vi "ZCR Find state by thresholds_temp.vi"(10 "Noise amplitude":dbl format="%.2p", 11 "Input Signal":waveform(dbl)[](graph)=[{"t0"=timestamp(3810040522.776 s since 1904-01-01), "dt"=0.0002, "Y"=array[5000 elements]}, {"t0"=timestamp(3810040522.777 s since 1904-01-01), "dt"=0.0002, "Y"=array[5000 elements]}]) -> (2 "SIN OFF Points":i32[](array[numeric]), 3 "SIN ON Points":i32[](array[numeric]))   [LabVIEW 2020, in "Library Commun.lvlib" / "Nodon_ZCR.lvclass"]
uses:
  Nodon_ZCR.lvclass
  <vilib>/Utility/miscctls.llb/LVRangeTypeDef.ctl
  <vilib>/measure/NI_MABase.lvlib
  <vilib>/Analysis/NI_AALPro.lvlib
panel:
  out "Graphe":dbl[](graph)
  in  "Point for zoom":i32
  out "Input Signal":waveform(dbl)[](graph)=[{"t0"=timestamp(3810040522.776 s since 1904-01-01), "dt"=0.0002, "Y"=array[5000 elements]}, {"t0"=timestamp(3810040522.777 s since 1904-01-01), "dt"=0.0002, "Y"=array[5000 elements]}]
  # "This VI Find the ON states and the OFF states based on a fix value\nNot to be used of ZCR control, due to the thresholds noise close to 0"
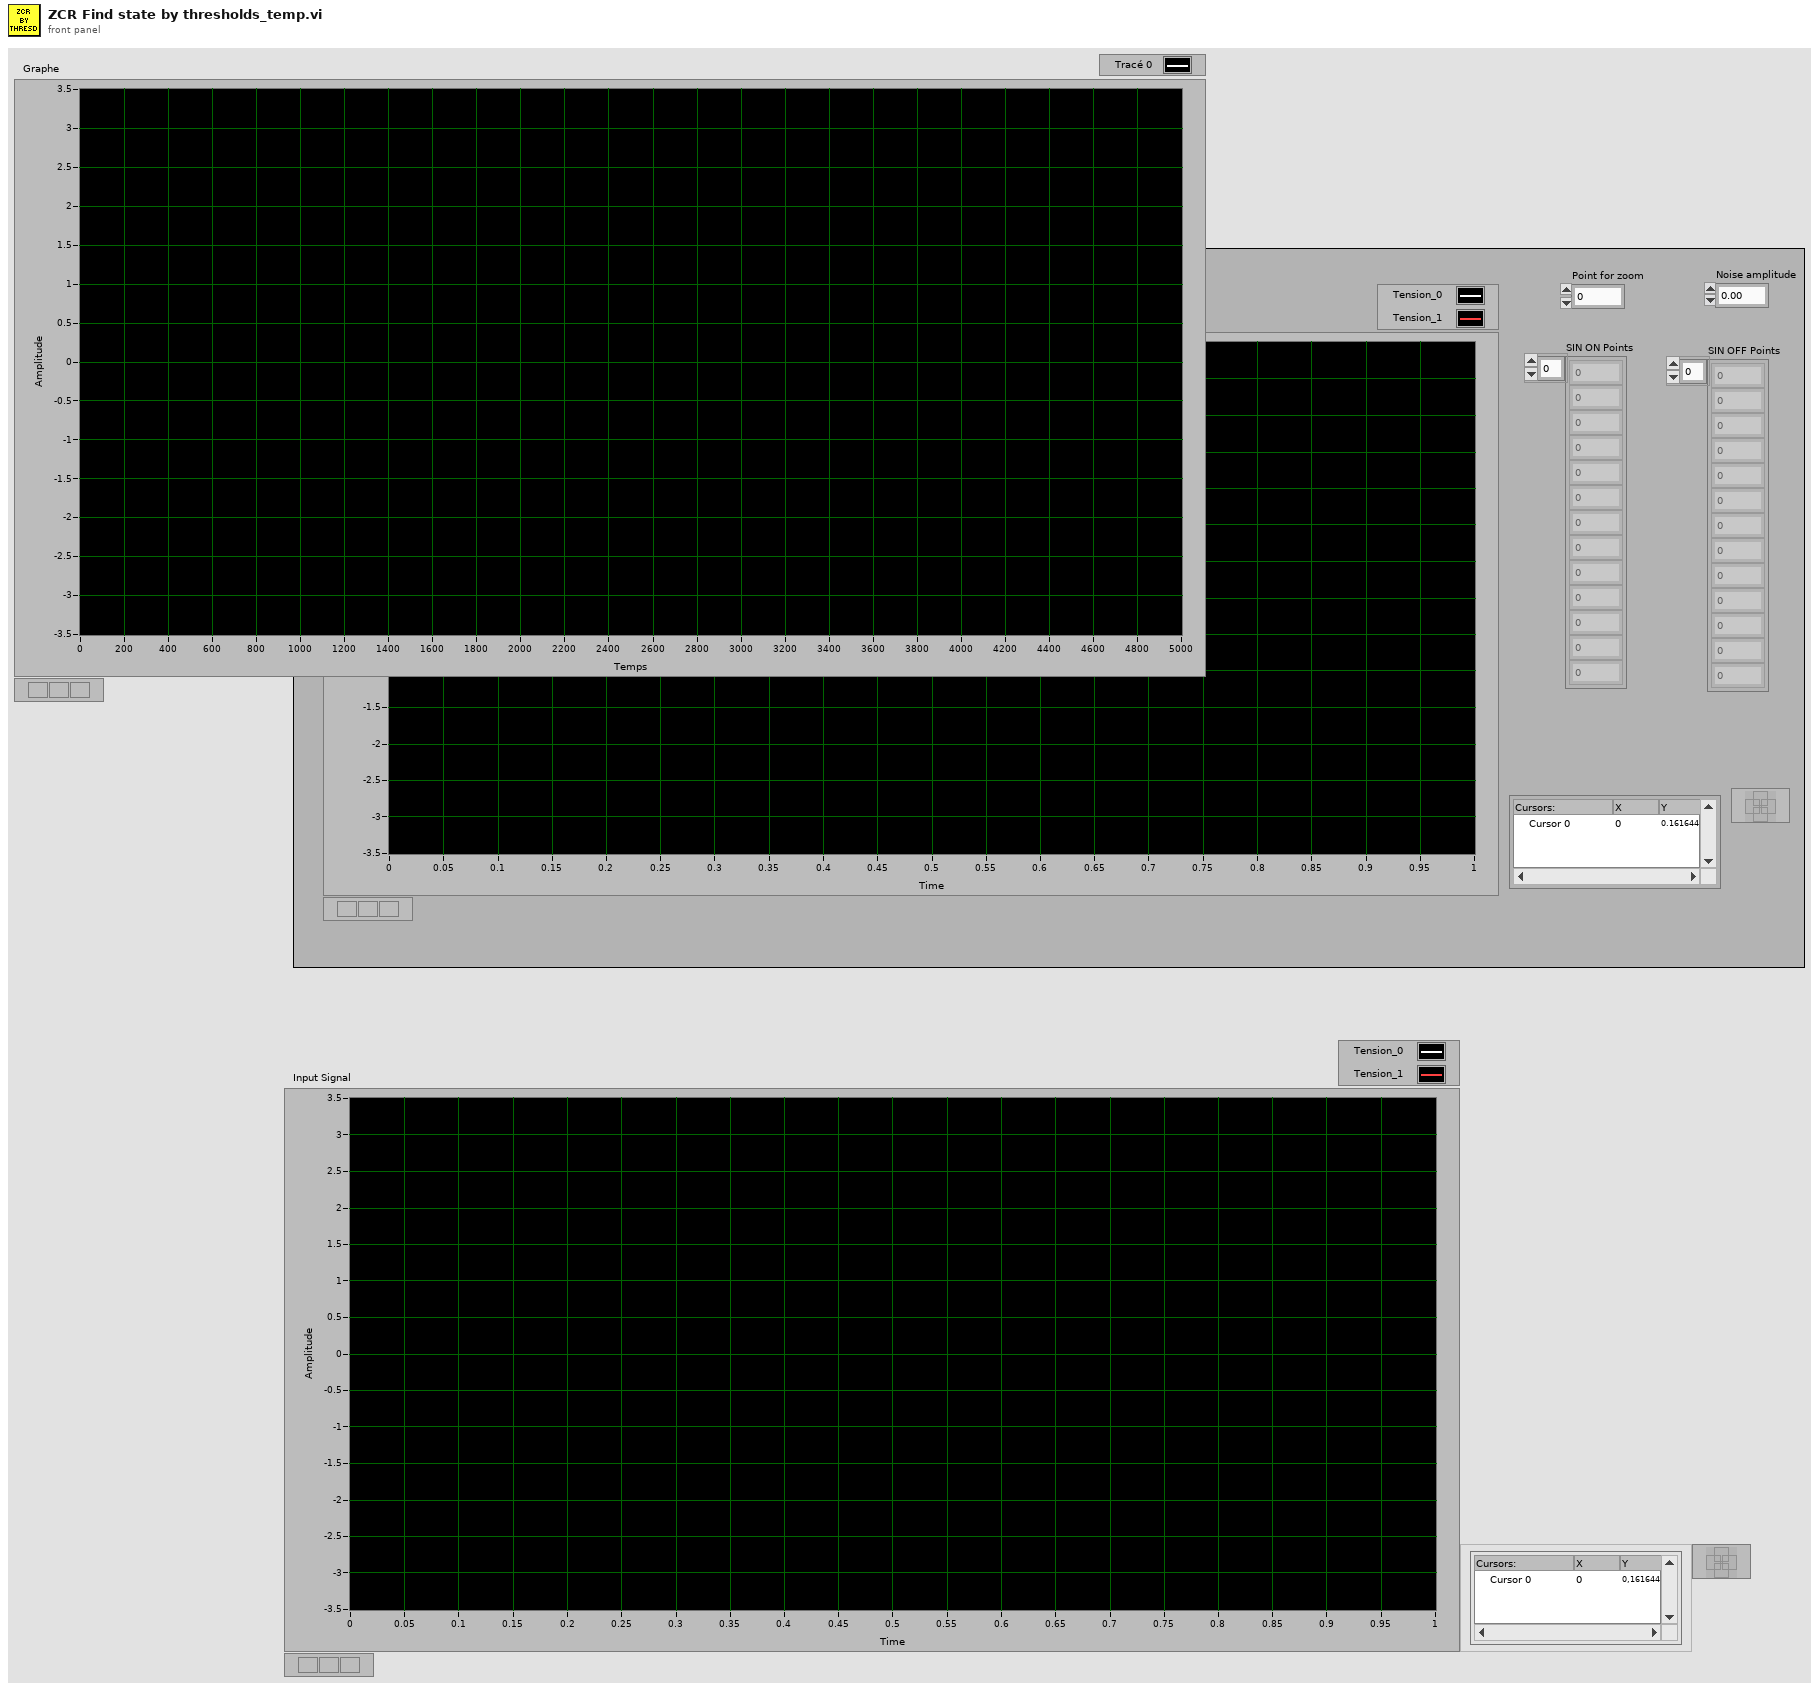
[diagram p1: front panel]
types:
  T1 = typedef "LVRangeTypeDef.ctl" = cluster{"Minimum":dbl, "Maximum":dbl, "Increment":dbl, "Minor Increment":dbl, "Start":dbl}
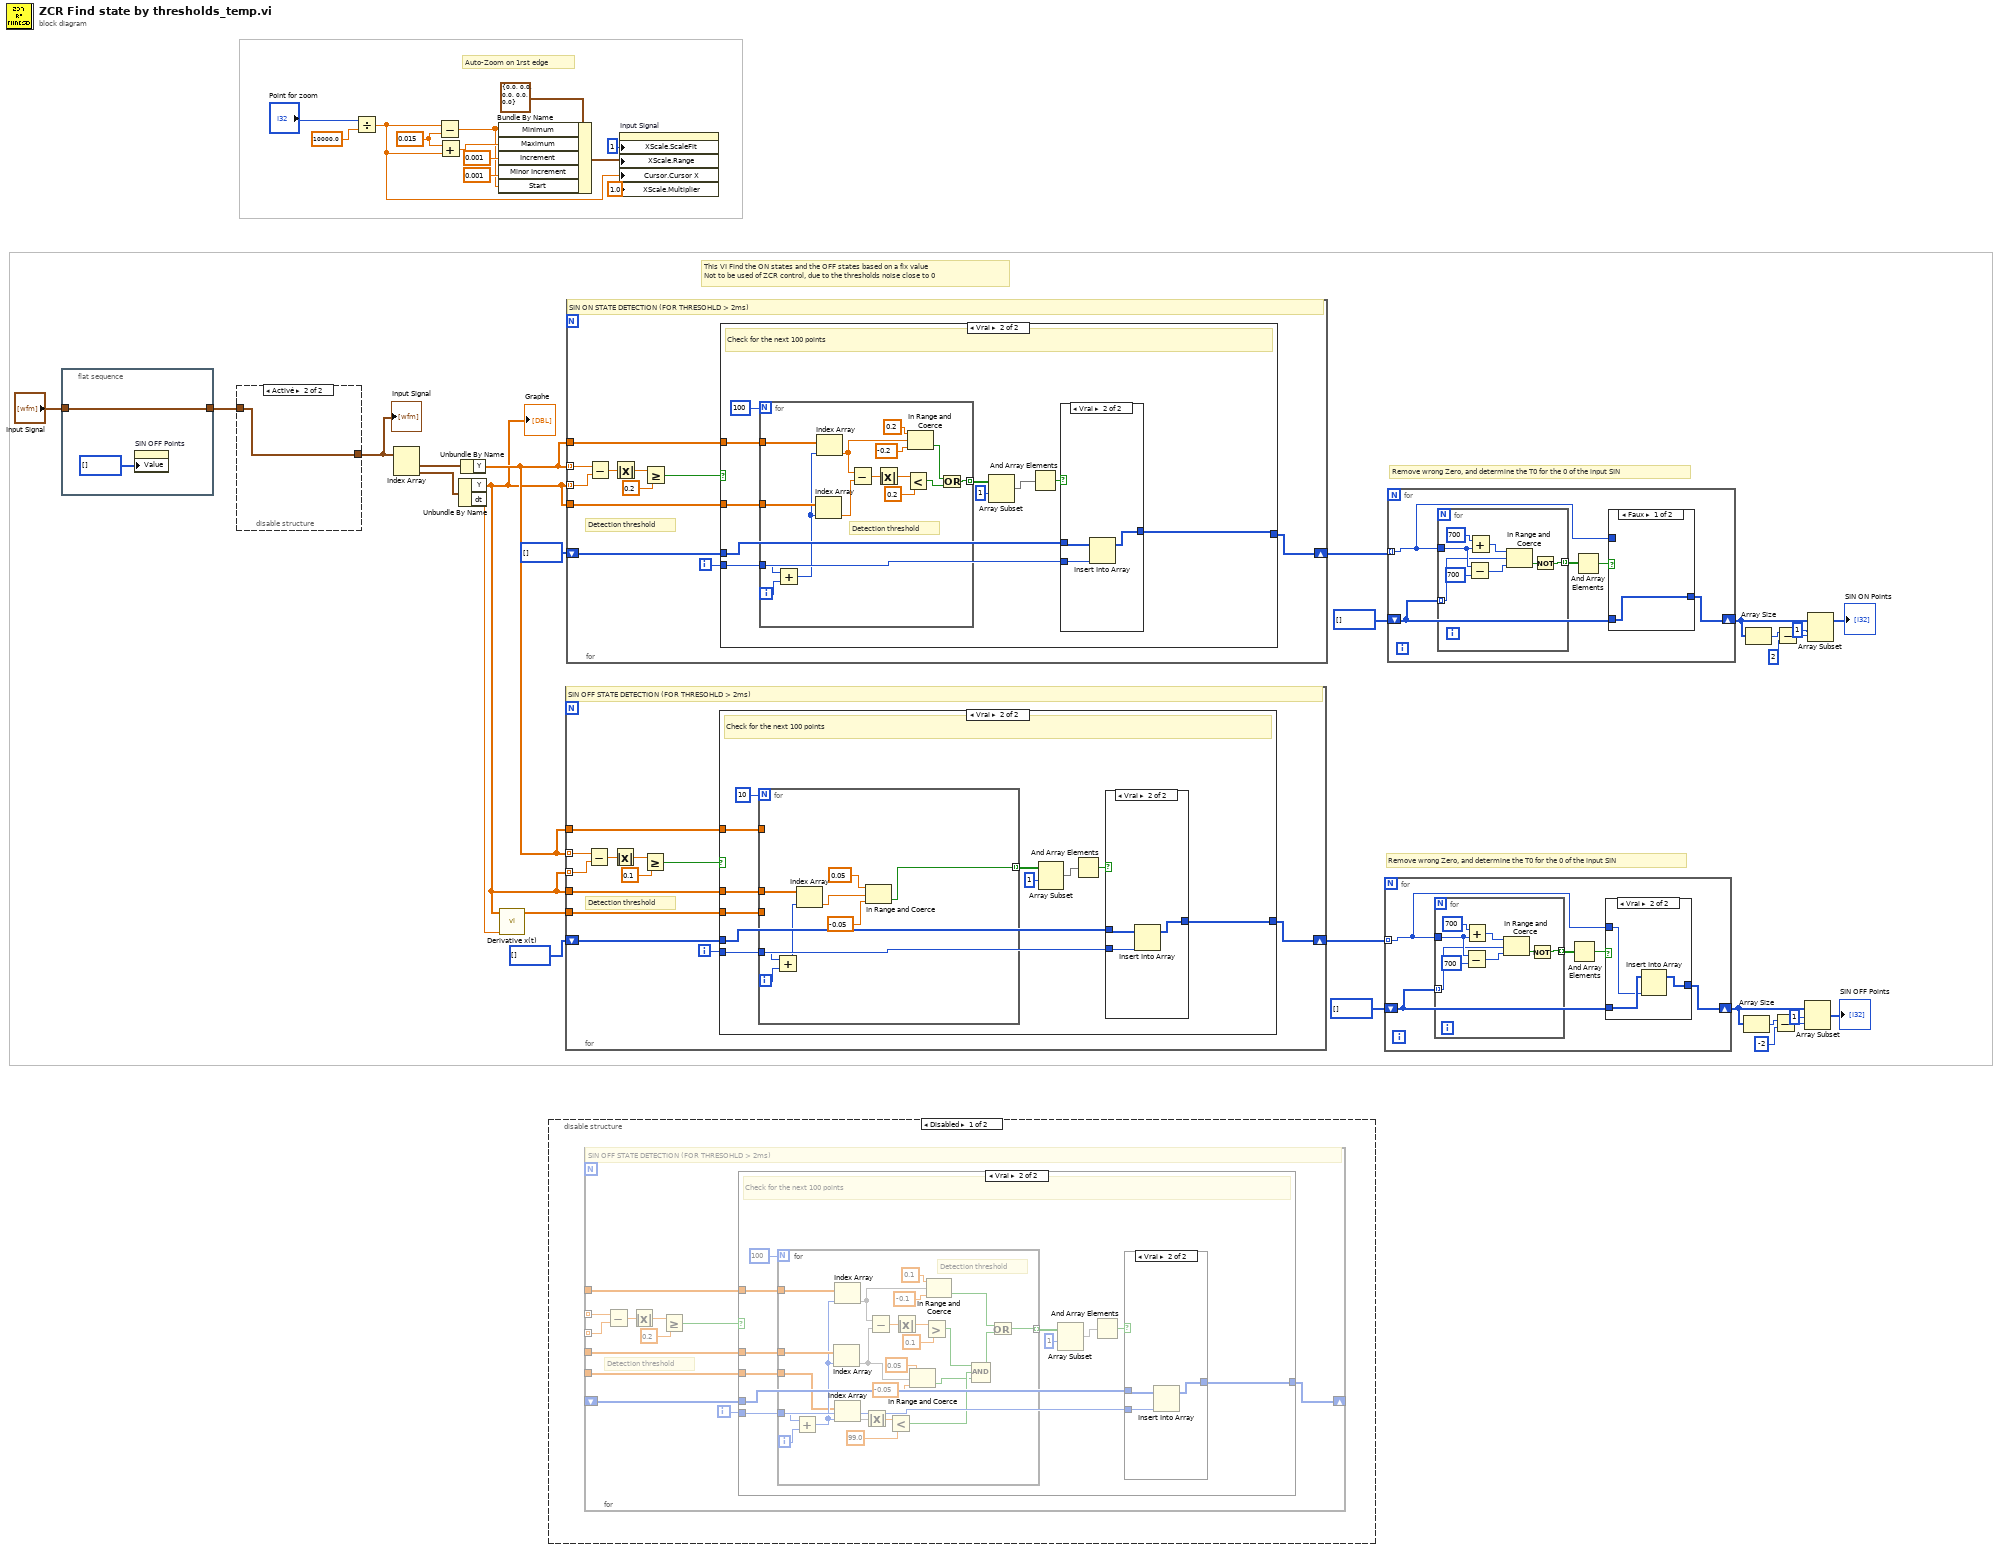
[diagram p0: block diagram]
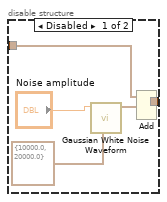
[diagram p2: hidden frame]
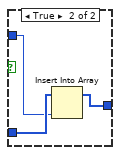
[diagram p6: hidden frame]
diagram:
  w34 = 0.015
  # "Remove wrong Zero, and determine the T0 for the 0 of the input SIN"
  # "Remove wrong Zero, and determine the T0 for the 0 of the input SIN"
  # "This VI Find the ON states and the OFF states based on a fix value\nNot to be used of ZCR control, due to the thresholds noise close to 0"
  # "Auto-Zoom on 1rst edge"
  n1 = flat-sequence {
    tunnel: "Input Signal" -> [w40]
    tunnel: [w40] -> w7
    frame #0 {
      n2 = property on="SIN OFF Points" class="Tabl (strict)"("Value"=i32[] []) -> ()  [unwired: 2 in, 2 out]
    }
  }
  n3 = disable-structure shown="Activé" {
    disable-tunnel: [w44 w47] -> w39
    disable-tunnel: w7 -> [w42 w47]
    frame Disabled {
      n4 = call <vilib>:"Gaussian White Noise Waveform.vi"("sampling info"=cluster{"Fs":dbl, "#s":dbl} {"Fs"=10000.0, "#s"=20000.0}, "standard deviation"="Noise amplitude") -> ("signal out"=w45:waveform(dbl))  [unwired: 8 in, 1 out]
      n5 = Add(1:w45, 2:w42) -> (0:w44:waveform(dbl)[])  [unwired: 1 in, 1 out]
    }
    frame Enabled {
    }
  }
  "Input Signal" <- w39
  n6 = Divide(x="Point for zoom", y=10000.0) -> (x/y=w25:dbl)
  n7 = Index Array(array=w39) -> (element #1=w38:waveform(dbl), element #2=w37:waveform(dbl))  [unwired: 2 in]
  n8 = Subtract(x=w25, y=w34) -> (x-y=w29:dbl)
  n9 = Add(x=w34, y=w25) -> (x+y=w32:dbl)
  n10 = Unbundle By Name(w37) -> ("Y"=w1:dbl[], "dt"=w3:dbl)
  "Graphe" <- w1
  n11 = Unbundle By Name(w38) -> ("Y"=w2:dbl[])
  n12 = Bundle By Name(cluster=T1 {"Minimum"=0.0, "Maximum"=0.0, "Increment"=0.0, "Minor Increment"=0.0, "Start"=0.0} ("X Scale.Range"), "Minimum"=w29, "Maximum"=w32, "Increment"=0.001, "Minor Increment"=0.001, "Start"=w29) -> (w28:T1)
  n13 = call <vilib>:"Derivative x(t).vi"("dt"=w3, "X"=w1) -> ("dX/dt"=w6:dbl[])  [unwired: 8 in, 1 out]
  n14 = disable-structure shown="Disabled" {
    frame Disabled {
      n15 = for {
        tunnel: _ -> [w59] mode=indexing
        tunnel: _ -> [w58] mode=indexing
        shift-right: [w51] -> _
        shift-left: _ -> [w53]
        tunnel: _ -> [w50]
        tunnel: _ -> [w49]
        tunnel: _ -> [w48]
        i -> [w52]
        # "Detection threshold"
        # "SIN OFF STATE DETECTION (FOR THRESOHLD > 2ms)"
        n16 = Subtract(x=w59, y=w58) -> (x-y=w57:dbl)
        n17 = Absolute Value(x=w57) -> (abs(x)=w56:dbl)
        n18 = Greater Or Equal?(x=w56, y=0.2) -> (x >= y?=w54:bool)
        n19 = case shown="Vrai" w54 {
          tunnel: w53 -> [w60 w67]
          tunnel: w52 -> [_ w66]
          tunnel: [w60 w65] -> w51
          tunnel: w50 -> [_ w69]
          tunnel: w49 -> [_ w70]
          tunnel: w48 -> [_ w61]
          frame False {
          }
          frame True {
            # "Check for the next 100 points"
            n20 = for {
              N: 100 -> [_]
              tunnel: w70 -> [w99]
              tunnel: w69 -> [w98]
              tunnel: w66 -> [w94]
              tunnel: [w84] -> w64 mode=indexing
              tunnel: w61 -> [w81]
              i -> [w82]
              # "Detection threshold"
              n21 = Add(x=w94, y=w82) -> (x+y=w90:i32)
              n22 = Index Array(array=w98, index=w90) -> (element=w76)
              n23 = Index Array(array=w99, index=w90) -> (element=w93)
              n24 = Index Array(array=w81, index=w90) -> (element=w89)
              n25 = Absolute Value(x=w89) -> (abs(x)=w80:dbl)
              n26 = Subtract(x=w93, y=w76) -> (x-y=w97:dbl)
              n27 = Less?(x=w80, y=99.0) -> (x < y?=w86:bool)
              n28 = Absolute Value(x=w97) -> (abs(x)=w96:dbl)
              n29 = In Range and Coerce(upper limit=0.05, x=w76, lower limit=-0.05) -> (In Range?=w77:bool)  [unwired: 1 out]
              n30 = Greater?(x=w96, y=0.1) -> (0:w87:bool)
              n31 = In Range and Coerce(upper limit=0.1, x=w93, lower limit=-0.1) -> (In Range?=w83:bool)  [unwired: 1 out]
              n32 = Compound Arithmetic op=AND(w87, w86, w77) -> (w85:bool)
              n33 = Or(x=w83, y=w85) -> (x .or. y?=w84:bool)
            }
            n34 = Array Subset(array=w64, index=1) -> (w63:bool[])  [unwired: 1 in]
            n35 = And Array Elements(Boolean array=w63) -> (logical AND=w68:bool)
            n36 = case shown="Vrai" w68 {
              tunnel: w67 -> [w72 w74]
              tunnel: w66 -> [_ w75]
              tunnel: [w72 w73] -> w65
              frame False {
              }
              frame True {
                n37 = Insert Into Array(array=w74, new element=w75) -> (w73:i32[])  [unwired: 1 in]
              }
            }
          }
        }
      }
    }
    frame Enabled {
    }
  }
  n38 = for {
    tunnel: w2 -> [w111] mode=indexing
    tunnel: w1 -> [w110] mode=indexing
    shift-right: [w103] -> w23
    shift-left: i32[] [] -> [w105]
    tunnel: w1 -> [w102]
    tunnel: w2 -> [w101]
    tunnel: w6 -> [w100]
    i -> [w104]
    # "Detection threshold"
    # "SIN OFF STATE DETECTION (FOR THRESOHLD > 2ms)"
    n39 = Subtract(x=w111, y=w110) -> (x-y=w109:dbl)
    n40 = Absolute Value(x=w109) -> (abs(x)=w108:dbl)
    n41 = Greater Or Equal?(x=w108, y=0.1) -> (x >= y?=w106:bool)
    n42 = case shown="Vrai" w106 {
      tunnel: w105 -> [w112 w119]
      tunnel: w104 -> [_ w118]
      tunnel: [w112 w117] -> w103
      tunnel: w102 -> [_ w121]
      tunnel: w101 -> [_ w122]
      tunnel: w100 -> [_ w115]
      frame False {
      }
      frame True {
        # "Check for the next 100 points"
        n43 = for {
          N: 10 -> [_]
          tunnel: w122 -> [_]
          tunnel: w121 -> [w130]
          tunnel: w118 -> [w135]
          tunnel: w115 -> [_]
          tunnel: [w131] -> w113 mode=indexing
          i -> [w134]
          n44 = Add(x=w135, y=w134) -> (x+y=w129:i32)
          n45 = Index Array(array=w130, index=w129) -> (element=w128:dbl)
          n46 = In Range and Coerce(upper limit=0.05, x=w128, lower limit=-0.05) -> (In Range?=w131:bool)  [unwired: 1 out]
        }
        n47 = Array Subset(array=w113, index=1) -> (w114:bool[])  [unwired: 1 in]
        n48 = And Array Elements(Boolean array=w114) -> (logical AND=w120:bool)
        n49 = case shown="Vrai" w120 {
          tunnel: w119 -> [w124 w126]
          tunnel: w118 -> [_ w127]
          tunnel: [w124 w125] -> w117
          frame False {
          }
          frame True {
            n50 = Insert Into Array(array=w126, new element=w127) -> (w125:i32[])  [unwired: 1 in]
          }
        }
      }
    }
  }
  n51 = for {
    tunnel: w2 -> [w146] mode=indexing
    tunnel: w1 -> [w145] mode=indexing
    shift-right: [w138] -> w21
    shift-left: i32[] [] -> [w140]
    tunnel: w1 -> [w137]
    tunnel: w2 -> [w136]
    i -> [w139]
    # "Detection threshold"
    # "SIN ON STATE DETECTION (FOR THRESOHLD > 2ms)"
    n52 = Subtract(x=w146, y=w145) -> (x-y=w144:dbl)
    n53 = Absolute Value(x=w144) -> (abs(x)=w143:dbl)
    n54 = Greater Or Equal?(x=w143, y=0.2) -> (x >= y?=w141:bool)
    n55 = case shown="Vrai" w141 {
      tunnel: w140 -> [w147 w153]
      tunnel: w139 -> [_ w152]
      tunnel: [w147 w151] -> w138
      tunnel: w137 -> [_ w155]
      tunnel: w136 -> [_ w156]
      frame False {
      }
      frame True {
        # "Check for the next 100 points"
        n56 = for {
          N: 100 -> [_]
          tunnel: w156 -> [w176]
          tunnel: w155 -> [w174]
          tunnel: w152 -> [w168]
          tunnel: [w162] -> w150 mode=indexing
          i -> [w175]
          # "Detection threshold"
          n57 = Add(x=w168, y=w175) -> (x+y=w173:i32)
          n58 = Index Array(array=w174, index=w173) -> (element=w169:dbl)
          n59 = Index Array(array=w176, index=w173) -> (element=w167:dbl)
          n60 = Subtract(x=w167, y=w169) -> (x-y=w172:dbl)
          n61 = Absolute Value(x=w172) -> (abs(x)=w171:dbl)
          n62 = Less?(x=w171, y=0.2) -> (x < y?=w164:bool)
          n63 = In Range and Coerce(upper limit=0.2, x=w167, lower limit=-0.2) -> (In Range?=w163:bool)  [unwired: 1 out]
          n64 = Or(x=w163, y=w164) -> (x .or. y?=w162:bool)
        }
        n65 = Array Subset(array=w150, index=1) -> (w149:bool[])  [unwired: 1 in]
        n66 = And Array Elements(Boolean array=w149) -> (logical AND=w154:bool)
        n67 = case shown="Vrai" w154 {
          tunnel: w153 -> [w158 w160]
          tunnel: w152 -> [_ w161]
          tunnel: [w158 w159] -> w151
          frame False {
          }
          frame True {
            n68 = Insert Into Array(array=w160, new element=w161) -> (w159:i32[])  [unwired: 1 in]
          }
        }
      }
    }
  }
  n69 = property on="Input Signal" class="GraphWF (strict)"("XScale.ScaleFit"=u8 1 ("X Scale.Scale Fit"), "XScale.Range"=w28, "Cursor.Cursor X"=w25, "XScale.Multiplier"=1.0 ("X Scale.Offset and Multiplier:Multiplier")) -> ()  [unwired: 2 in, 2 out]
  n70 = for {
    tunnel: w23 -> [w179] mode=indexing
    shift-right: [w180] -> w15
    shift-left: i32[] [] -> [w181]
    n71 = for {
      tunnel: w179 -> [w189]
      tunnel: w181 -> [w186] mode=indexing
      tunnel: [w187] -> w178 mode=indexing
      n72 = Subtract(x=w189, y=700) -> (x-y=w190:i32)
      n73 = Add(x=700, y=w189) -> (x+y=w191:i32)
      n74 = In Range and Coerce(upper limit=w191, x=w186, lower limit=w190) -> (In Range?=w188:bool)  [unwired: 1 out]
      n75 = Not(x=w188) -> (.not. x?=w187:bool)
    }
    n76 = And Array Elements(Boolean array=w178) -> (logical AND=w177:bool)
    n77 = case shown="Vrai" w177 {
      tunnel: w181 -> [w182 w184]
      tunnel: [w182 w185] -> w180
      tunnel: w179 -> [_ w183]
      frame False {
      }
      frame True {
        n78 = Insert Into Array(array=w184, new element=w183) -> (w185:i32[])  [unwired: 1 in]
      }
    }
  }
  n79 = for {
    tunnel: w21 -> [w196] mode=indexing
    shift-right: [w197] -> w18
    shift-left: i32[] [] -> [w198]
    n80 = for {
      tunnel: w196 -> [w206]
      tunnel: w198 -> [w203] mode=indexing
      tunnel: [w204] -> w195 mode=indexing
      n81 = Subtract(x=w206, y=700) -> (x-y=w207:i32)
      n82 = Add(x=700, y=w206) -> (x+y=w208:i32)
      n83 = In Range and Coerce(upper limit=w208, x=w203, lower limit=w207) -> (In Range?=w205:bool)  [unwired: 1 out]
      n84 = Not(x=w205) -> (.not. x?=w204:bool)
    }
    n85 = And Array Elements(Boolean array=w195) -> (logical AND=w194:bool)
    n86 = case shown="Faux" w194 {
      tunnel: w198 -> [w199 w201]
      tunnel: [w199 w202] -> w197
      tunnel: w196 -> [_ w200]
      frame False {
      }
      frame True {
        n87 = Insert Into Array(array=w201, new element=w200) -> (w202:i32[])  [unwired: 1 in]
      }
    }
  }
  n88 = Array Size(array=w15) -> (size(s)=w9:i32)
  n89 = Array Size(array=w18) -> (size(s)=w11:i32)
  n90 = Subtract(x=w9, y=-2) -> (x-y=w16:i32)
  n91 = Subtract(x=w11, y=2) -> (x-y=w17:i32)
  n92 = Array Subset(array=w15, index=1, length=w16) -> (→"SIN OFF Points":i32[])
  n93 = Array Subset(array=w18, index=1, length=w17) -> (→"SIN ON Points":i32[])
